vi "SailSetSuggestions.vi"() -> ()   [LabVIEW 2012]
doc: "Returns suggestions for the sail positions (0-1) based on the current state of the boat. This outputs a number of suggestions, which are blended in the arbiter in Act.\n\nInputs: relative wind angle, degree of luffing, rudder force, the direction of the boat, and the desired direction of the boat.\n\nAngles should follow the Sailbot standard of 0 East and CCW increase, except for Relative Wind. Velocities should be in (m/s). RudderForce and DegreeOfLuffing are not settled yet, but 0-1 would be reasonable.\n\nEric Schneider and Bonnie Ishiguro, Jan. 2014"
uses:
  Data/TypeDefs/Sail Set Suggestions.ctl
  Data/TypeDefs/Rudder Set Suggestions.ctl
  Data/TypeDefs/MB Think to Act Bundled Sail Commands.ctl
panel:
  out "SailSuggestionToMB-ACTArbiter":T1 {"SailByWindLookup"."MainSailSuggestion" min=0.0 max=1.0; "SailByWindLookup"."JibSailSuggestion" min=0.0 max=1.0; "SailsByTurningBoat"."MainSailSuggestion" min=0.0 max=1.0; "SailsByTurningBoat"."JibSailSuggestion" min=0.0 max=1.0; "SailByTurtleMode"."MainSailSuggestion" min=0.0 max=1.0; "SailByTurtleMode"."JibSailSuggestion" min=0.0 max=1.0; "RudderByTurtleMode" min=-1.0 max=1.0; "SailsByReducingLuffing"."MainSailSuggestion" min=0.0 max=1.0; "SailsByReducingLuffing"."JibSailSuggestion" min=0.0 max=1.0; "SailsByBalancingRudder"."MainSailSuggestion" min=0.0 max=1.0; "SailsByBalancingRudder"."JibSailSuggestion" min=0.0 max=1.0; "TackManeuverSails"."MainSailSuggestion" min=0.0 max=1.0; "TackManeuverSails"."JibSailSuggestion" min=0.0 max=1.0; "TackManeuverRudder" min=-1.0 max=1.0; "JibeManeuverSails"."MainSailSuggestion" min=0.0 max=1.0; "JibeManeuverSails"."JibSailSuggestion" min=0.0 max=1.0; "JibeManeuverRudder" min=-1.0 max=1.0}
  in  "BoatSpeed":dbl
  in  "WindSpeed":dbl
  in  "AbsoluteWindAngle":dbl
  in  "DesiredHeading":dbl
  in  "RobotHeading":dbl
  in  "RudderForce":dbl
  in  "DegreeOfLuffing":dbl
  in  "RelativeWindAngle":dbl
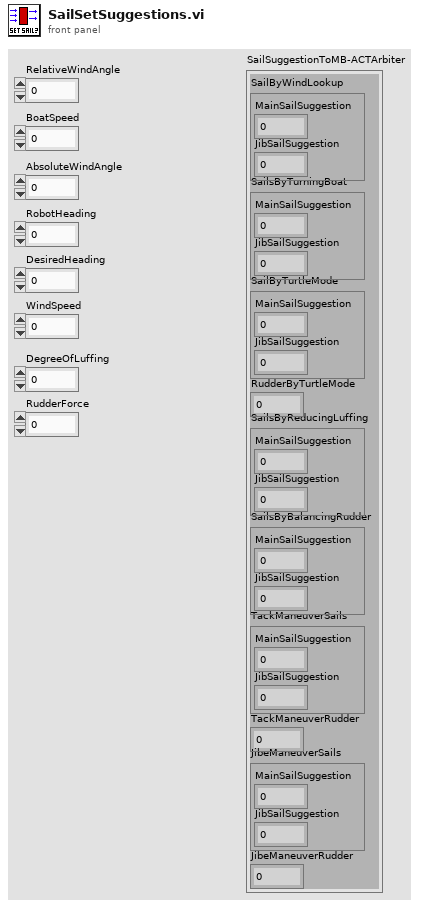
[diagram p1: front panel]
types:
  T1 = typedef "MB Think to Act Bundled Sail Commands.ctl" = cluster{"SailByWindLookup":T2, "SailsByTurningBoat":T2, "SailByTurtleMode":T2, "RudderByTurtleMode":T3, "SailsByReducingLuffing":T2, "SailsByBalancingRudder":T2, "TackManeuverSails":T2, "TackManeuverRudder":T3, "JibeManeuverSails":T2, "JibeManeuverRudder":T3}
  T2 = typedef "Sail Set Suggestions.ctl" = cluster{"MainSailSuggestion":dbl, "JibSailSuggestion":dbl}
  T3 = typedef "Rudder Set Suggestions.ctl" = dbl
  T4 = cluster{"SailByWindLookup":T2, "SailsByTurningBoat":T2, "SailByTurtleMode":T2, "RudderByTurtleMode":T3, "SailsByReducingLuffing":T2, "SailsByBalancingRudder":T2, "TackManeuverSails":T2, "TackManeuverRudder":T3, "JibeManeuverSails":T2, "JibeManeuverRudder":T3}
  T5 = cluster{"BoatVelocityInY":dbl, "BoatVelocityInX":dbl}
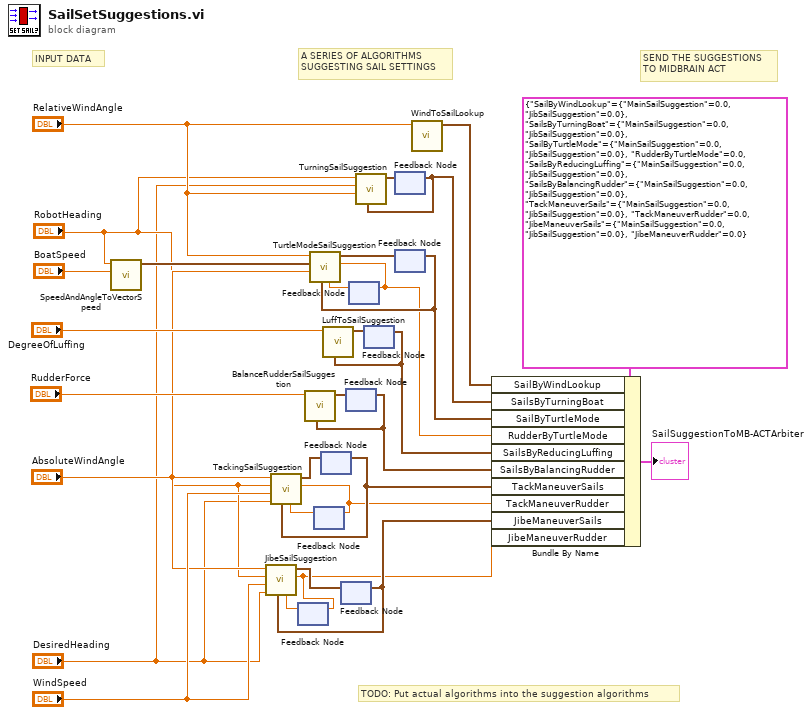
[diagram p0: block diagram]
diagram:
  # "SEND THE SUGGESTIONS\nTO MIDBRAIN ACT"
  # "A SERIES OF ALGORITHMS\nSUGGESTING SAIL SETTINGS"
  # "INPUT DATA"
  # "TODO: Put actual algorithms into the suggestion algorithms"
  n1 = call "SpeedAndAngleToVectorSpeed.vi"("BoatSpeed (m/s)"="BoatSpeed", "RobotHeading (deg)"="RobotHeading") -> ("BoatVectorVelocity"=w5:T5)  [unwired: 9 in]
  n2 = feedback #1() -> (w21:T3)  [unwired: 1 in]
  n3 = feedback #2() -> (w19:T3)  [unwired: 1 in]
  n4 = feedback #3() -> (w12:T2)  [unwired: 1 in]
  n5 = call "TackingSailSuggestion.vi"("OLD Suggested Rudder Setpoint"=w19, "OLD Suggested Sail Setpoints"=w12, "DesiredHeading"="DesiredHeading", "WindSpeed"="WindSpeed", "RobotHeading"="RobotHeading", "AbsoluteWindAngle"="AbsoluteWindAngle") -> ("Suggested Rudder Setpoint"=w7:T3, "Suggested Sail Setpoints"=w20:T2)  [unwired: 4 in]
  n6 = feedback-in #2(w7) -> ()
  n7 = feedback-in #3(w20) -> ()
  n8 = feedback #4() -> (w11:T2)  [unwired: 1 in]
  n9 = call "JibeSailSuggestion.vi"("OLD Suggested Rudder Setpoint"=w21, "OLD Suggested Sail Setpoints"=w11, "DesiredHeading"="DesiredHeading", "WindSpeed"="WindSpeed", "RobotHeading"="RobotHeading", "AbsoluteWindAngle"="AbsoluteWindAngle") -> ("Suggested Rudder Setpoint"=w1:T3, "Suggested Sail Setpoints"=w22:T2)  [unwired: 4 in]
  n10 = feedback-in #1(w1) -> ()
  n11 = feedback-in #4(w22) -> ()
  n12 = feedback #5() -> (w8:T2)  [unwired: 1 in]
  n13 = call "BalanceRudderSailSuggestion.vi"("OLD Suggested Sail Setpoints"=w8, "ForceOnRudder"="RudderForce") -> ("Suggested Sail Setpoints"=w17:T2)  [unwired: 9 in]
  n14 = feedback-in #5(w17) -> ()
  n15 = feedback #6() -> (w23:T3)  [unwired: 1 in]
  n16 = feedback #7() -> (w9:T2)  [unwired: 1 in]
  n17 = call "LuffToSailSuggestion.vi"("OLD Suggested Sail Setpoints"=w9, "DegreeOfLuffing"="DegreeOfLuffing") -> ("Suggested Sail Setpoints"=w18:T2)  [unwired: 9 in]
  n18 = feedback-in #7(w18) -> ()
  n19 = feedback #8() -> (w15:T2)  [unwired: 1 in]
  n20 = call "TurningSailSuggestion.vi"("Old Suggested Sail Setpoints"=w15, "RelativeWindAngle"="RelativeWindAngle", "DesiredHeading"="DesiredHeading", "RobotHeading"="RobotHeading") -> ("Suggested Sail Setpoints"=w25:T2)  [unwired: 7 in]
  n21 = feedback-in #8(w25) -> ()
  n22 = feedback #9() -> (w14:T2)  [unwired: 1 in]
  n23 = call "TurtleModeSailSuggestion.vi"("OLD Suggested Rudder Setpoint"=w23, "OLD Suggested Sail Setpoints"=w14, "AbsoluteWindAngle"="AbsoluteWindAngle", "BoatVectorVelocity"=w5, "RelativeWindAngle"="RelativeWindAngle") -> ("Suggested Rudder Setpoint"=w13:T3, "Suggested Sail Setpoints"=w24:T2)  [unwired: 5 in]
  n24 = feedback-in #6(w13) -> ()
  n25 = feedback-in #9(w24) -> ()
  n26 = call "WindToSailLookup.vi"("RelativeWindAngle"="RelativeWindAngle") -> ("Suggested Sail Setpoints"=w16:T2)  [unwired: 10 in]
  n27 = Bundle By Name(cluster=T4 {"SailByWindLookup"={"MainSailSuggestion"=0.0, "JibSailSuggestion"=0.0}, "SailsByTurningBoat"={"MainSailSuggestion"=0.0, "JibSailSuggestion"=0.0}, "SailByTurtleMode"={"MainSailSuggestion"=0.0, "JibSailSuggestion"=0.0}, "RudderByTurtleMode"=0.0, "SailsByReducingLuffing"={"MainSailSuggestion"=0.0, "JibSailSuggestion"=0.0}, "SailsByBalancingRudder"={"MainSailSuggestion"=0.0, "JibSailSuggestion"=0.0}, "TackManeuverSails"={"MainSailSuggestion"=0.0, "JibSailSuggestion"=0.0}, "TackManeuverRudder"=0.0, "JibeManeuverSails"={"MainSailSuggestion"=0.0, "JibSailSuggestion"=0.0}, "JibeManeuverRudder"=0.0} ("input cluster"), "SailByWindLookup"=w16, "SailsByTurningBoat"=w15, "SailByTurtleMode"=w14, "RudderByTurtleMode"=w13, "SailsByReducingLuffing"=w9, "SailsByBalancingRudder"=w8, "TackManeuverSails"=w12, "TackManeuverRudder"=w7, "JibeManeuverSails"=w11, "JibeManeuverRudder"=w1) -> (→"SailSuggestionToMB-ACTArbiter":T4)
